vi "Write Handle.vi"(8 "error in (no error)":errorcluster, 10 "Handle":u64, 11 "SSL in":refnum<class "SSL.lvclass">) -> (0 "error out":errorcluster, 3 "SSL out":refnum<class "SSL.lvclass">)   [LabVIEW 2013, in "SSL_Lib.lvlib" / "SSL.lvclass"]
uses:
  SSL.lvclass
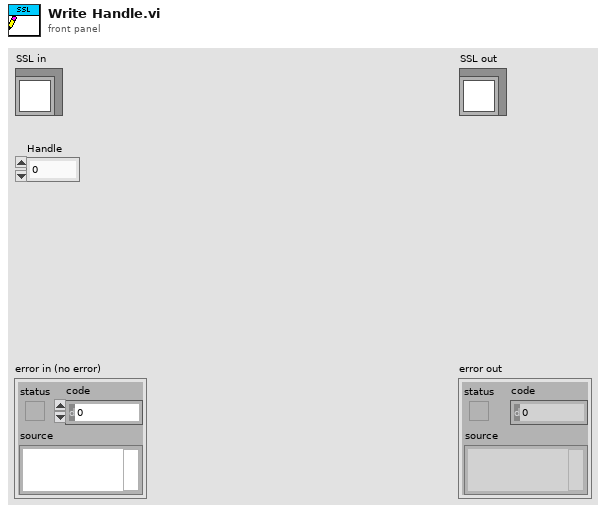
[diagram p1: front panel]
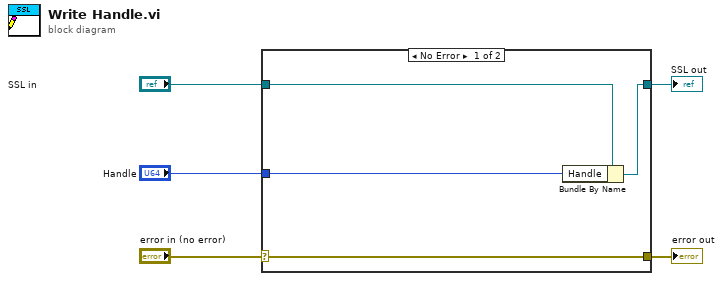
[diagram p0: block diagram]
diagram:
  n1 = case shown="No Error" "error in (no error)" {
    selector: "error in (no error)" -> [w9 w10]
    tunnel: [w9 w10] -> w4
    tunnel: [w7 w11] -> w2
    tunnel: "SSL in" -> [w8 w11]
    tunnel: "Handle" -> [w6 _]
    frame No Error {
      n2 = Bundle By Name(cluster=w8, "Handle"=w6) -> (w7:refnum<class "SSL.lvclass">)
    }
    frame Error {
    }
  }
  "error out" <- w4
  "SSL out" <- w2
